vi "G#Debugger_RemoveObject.vi"(0 "Objects dvr":refnum<data-value>, 1 "ObjectInfo":T2, 5 "error in (no error)":errorcluster) -> (16 "Elements":T1, 19 "error out":errorcluster)   [LabVIEW 2017, in "G#Debugger.lvlib"]
uses:
  G#Debugger.lvlib
  G#Object/utils/G#Object_ClassInfoType.ctl
  G#Object/G#Object.lvclass
  G#Object/utils/G#Object_ObjectInfoType.ctl
  G#Object/utils/G#Object_CreateMethod.ctl
  G#Debugger_TreeElement.ctl
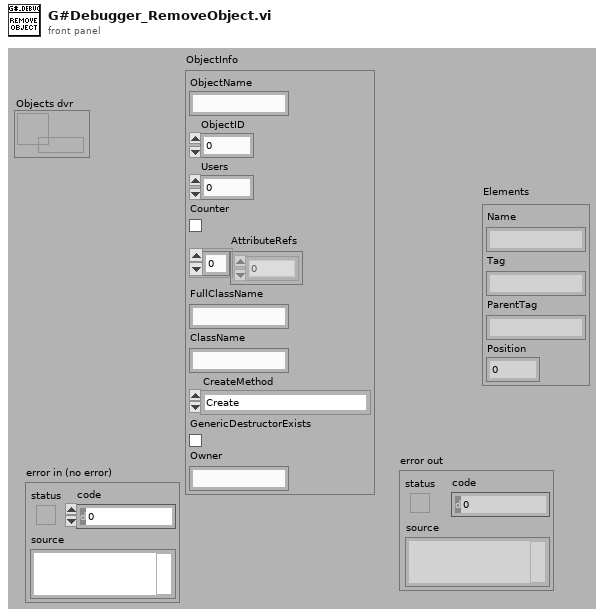
[diagram p1: front panel]
types:
  T1 = typedef "G#Debugger.lvlib/G#Debugger_TreeElement.ctl" = cluster{"Name":string, "Tag":string, "ParentTag":string, "Position":i32}
  T2 = typedef "G#Object.lvclass/G#Object_ObjectInfoType.ctl" = cluster{"ObjectName":string, "ObjectID":u32, "Users":i32, "Counter":bool, "AttributeRefs":u32[], "FullClassName":string, "ClassName":string, "CreateMethod":T3, "GenericDestructorExists":bool, "Owner":string}
  T3 = typedef "G#Object.lvclass/G#Object_CreateMethod.ctl" = enum16{"Create", "Create or look up existing", "Look up existing"}
  T4 = typedef "G#Object.lvclass/G#Object_ClassInfoType.ctl" = cluster{"ClassName":string, "ObjectInfo":T2[], "ObjectRefs":refnum<class "G#Object.lvclass">[], "TypeRef":refnum<class "G#Object.lvclass">}
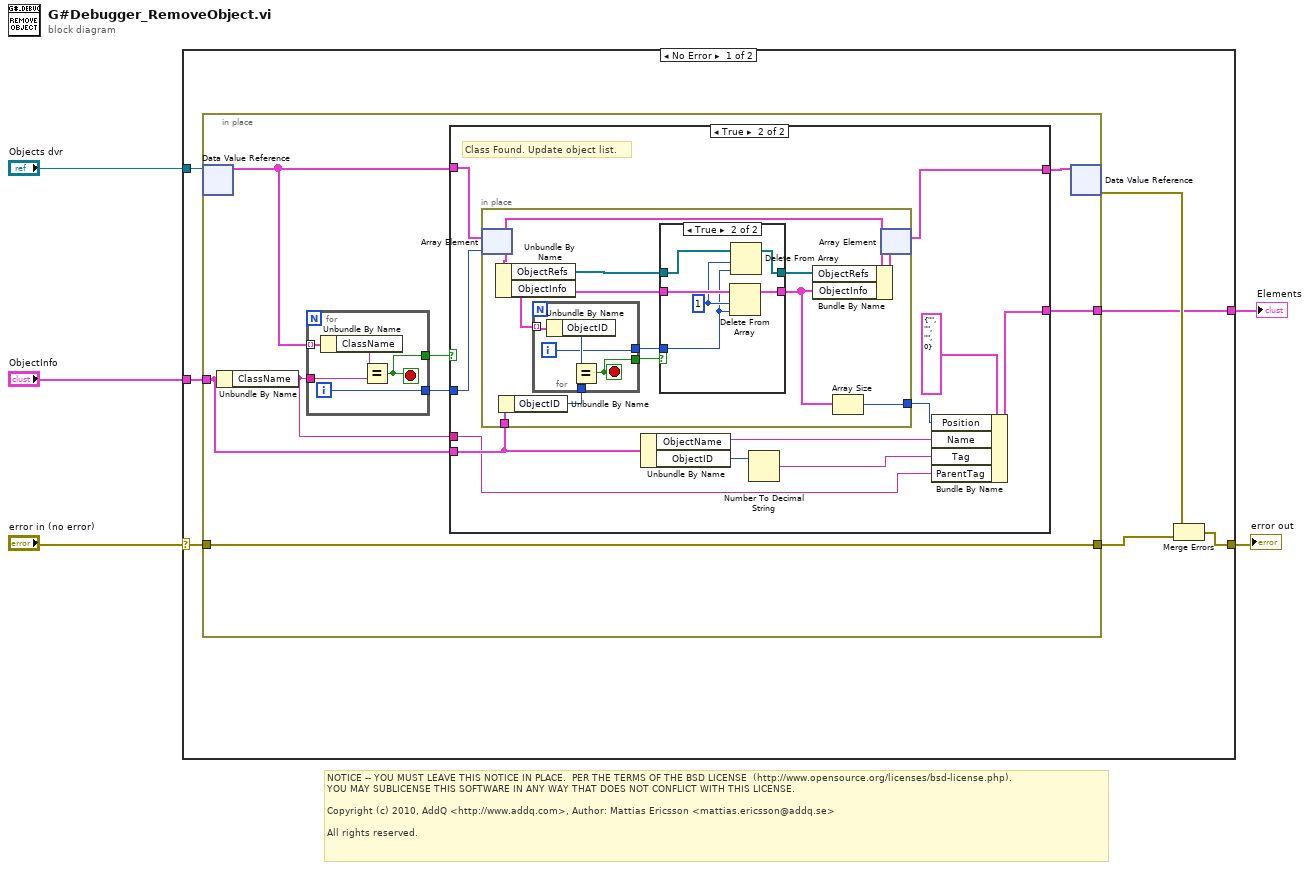
[diagram p0: block diagram]
diagram:
  # "NOTICE -- YOU MUST LEAVE THIS NOTICE IN PLACE.  PER THE TERMS OF THE BSD LICENSE  (http://www.opensource.org/licenses/bsd-license.php).\nYOU MAY SUBLICENSE THIS SOFTWARE IN ANY WAY THAT DOES NOT CONFLICT WITH THIS LICENSE.\n\nCopyright (c) 2010, AddQ <http://www.addq.com>, Author: Mattias Ericsson <mattias.ericsson@addq.se>\n\nAll rights reserved."
  n1 = case shown="No Error" "error in (no error)" {
    selector: "error in (no error)" -> [w12 w62]
    tunnel: [w10 w62] -> w4
    tunnel: "Objects dvr" -> [w11 _]
    tunnel: "ObjectInfo" -> [w8 _]
    tunnel: [w6 _] -> w1
    frame No Error {
      n2 = in-place {
        in-place-border: w12 -> [w14]
        in-place-border: w8 -> [w17]
        in-place-border: [w14] -> w7
        in-place-border: [w13] -> w6
        n3 = in-place-dvr #1(w11) -> (w19:T4[])  [unwired: 1 out]
        n4 = Unbundle By Name(w17) -> ("ClassName"=w15:string)
        n5 = for {
          tunnel: w19 -> [w61] mode=indexing
          tunnel: w15 -> [w59]
          tunnel: [w58] -> w18
          tunnel: [w57] -> w20
          i -> [w58]
          stop <- w57 stop-if-true
          n6 = Unbundle By Name(w61) -> ("ClassName"=w60:string)
          n7 = Equal?(x=w60, y=w59) -> (x = y?=w57:bool)
        }
        n8 = case shown="True" w20 {
          tunnel: w19 -> [w21 w32]
          tunnel: w18 -> [_ w30]
          tunnel: w17 -> [_ w28]
          tunnel: [w21 w31] -> w16
          tunnel: w15 -> [_ w24]
          tunnel: [_ w22] -> w13
          frame False {
            # "Class not found, nothing to delete"
          }
          frame True {
            # "Class Found. Update object list."
            n9 = in-place {
              in-place-border: w28 -> [w41]
              in-place-border: [w35] -> w23
              n10 = in-place-array #2(w32, w30) -> (w43:T4)
              n11 = Unbundle By Name(w43) -> ("ObjectRefs"=w34:refnum<class "G#Object.lvclass">[], "ObjectInfo"=w38:T2[])
              n12 = Unbundle By Name(w41) -> ("ObjectID"=w40:u32)
              n13 = for {
                tunnel: w38 -> [w56] mode=indexing
                tunnel: w40 -> [w54]
                tunnel: [w53] -> w39
                tunnel: [w52] -> w37
                i -> [w52]
                stop <- w53 stop-if-true
                n14 = Unbundle By Name(w56) -> ("ObjectID"=w55:u32)
                n15 = Equal?(x=w55, y=w54) -> (x = y?=w53:bool)
              }
              n16 = case shown="True" w39 {
                tunnel: w38 -> [w45 w51]
                tunnel: [w45 w50] -> w36
                tunnel: w37 -> [_ w46]
                tunnel: w34 -> [w44 w49]
                tunnel: [w44 w48] -> w33
                frame False {
                  # "Not found"
                }
                frame True {
                  w47 = 1 ("length")
                  n17 = Delete From Array(array=w51, length=w47, index=w46) -> (array with subset deleted=w50:T2[])  [unwired: 1 out]
                  n18 = Delete From Array(array=w49, length=w47, index=w46) -> (array with subset deleted=w48:refnum<class "G#Object.lvclass">[])  [unwired: 1 out]
                }
              }
              n19 = Bundle By Name(cluster=w43, "ObjectRefs"=w33, "ObjectInfo"=w36) -> (w42:T4)
              n20 = Array Size(array=w36) -> (size(s)=w35:i32)
              n21 = in-place-array #2(w42) -> (w31:T4[])  [unwired: 1 out]
            }
            n22 = Unbundle By Name(w28) -> ("ObjectName"=w27:string, "ObjectID"=w26:u32)
            n23 = Number To Decimal String(number=w26) -> (decimal integer string=w25:string)  [unwired: 1 in]
            n24 = Bundle By Name(cluster=T1 {"Name"="", "Tag"="", "ParentTag"="", "Position"=0} ("Cluster"), "Position"=w23, "Name"=w27, "Tag"=w25, "ParentTag"=w24) -> (w22:T1)
          }
        }
        n25 = in-place-dvr #1(w16) -> (w9:errorcluster)  [unwired: 1 out]
      }
      n26 = Merge Errors(w9, w7) -> (w10:errorcluster)
    }
    frame Error {
    }
  }
  "error out" <- w4
  "Elements" <- w1
